vi "toULong64Scalar.vi"(2 "value_in":u8[](array[numeric]), 3 "dim_y":i32, 4 "dim_x":i32) -> (0 "setpoint":u64, 1 "value":u64)   [LabVIEW 2014, in "tango.lvlib"]
uses:
  tango.lvlib
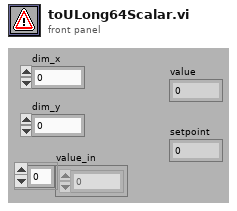
[diagram p1: front panel]
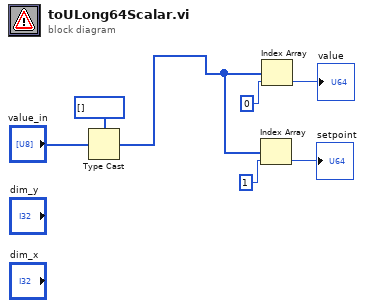
[diagram p0: block diagram]
diagram:
  n1 = Type Cast(type=u64[] [], x="value_in") -> (*(type *) &x=w1:u64[])
  n2 = Index Array(array=w1, index=1 ("indice")) -> (element=→"setpoint":u64)
  n3 = Index Array(array=w1, index=0 ("indice")) -> (element=→"value":u64)
